vi "GLB_AIs.vi"() -> ()   [LabVIEW 2014, in "PLS Acquisition.lvlib"]
uses:
  PLS Acquisition.lvlib
panel:
  in  "AIs":T1
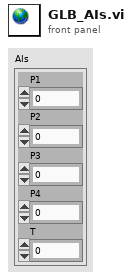
[diagram p1: front panel]
types:
  T1 = cluster{"P1":dbl, "P2":dbl, "P3":dbl, "P4":dbl, "T":dbl}
diagram:
